vi "setSamplingMode.vi"(8 "error in (no error)":errorcluster, 10 "Fs Mode":T1, 11 "Instrument.Lockin in":refnum<class "Instrument.Lockin.lvclass">) -> (0 "error out":errorcluster, 3 "Instrument.Lockin out":refnum<class "Instrument.Lockin.lvclass">)   [LabVIEW 2019, in "Instrument.Lockin.lvclass"]
doc: "API to put lockin into IV mode.\n\nIf address=\"\", this API reads from localhost\nIf address is remote lockin, you need to add this computer to allowed whitelist on the lockin computer you are trying to access."
uses:
  Instrument.Lockin.lvclass
  Instrument.DAQ/Typedefs/DAQ.Sampling.Fs Mode--enum.ctl
  C:/Program Files (x86)/National Instruments/LabVIEW 2019/user.lib/LevyLab/Instrument Framework/SMOs/Instrument/Instrument.lvclass
  Typedefs/API/Lockin.Commands--Enum.ctl
  <userlib>/LevyLab/Instrument Framework/SMOs/Instrument/Instrument.lvclass/Instrument.ctl
  08458c74-1ef2-45d6-87a0-b6580aa97565.vi
  08458c74-1ef2-45d6-87a0-b6580aa97565.vi/21b8891c-77eb-44a0-bd46-0f361e5e9657.vi
  08458c74-1ef2-45d6-87a0-b6580aa97565.vi/21b8891c-77eb-44a0-bd46-0f361e5e9657.vi/e1bdb0cf-b8bc-43bb-a77e-4995ee286623.vi
  <userlib>/LevyLab/Instrument Framework/SMOs/Instrument/API/Send and Receive.vi
  08458c74-1ef2-45d6-87a0-b6580aa97565.vi/21b8891c-77eb-44a0-bd46-0f361e5e9657.vi/e1bdb0cf-b8bc-43bb-a77e-4995ee286623.vi/20487861-9e4a-4482-b9dd-50cdbc220220.vi
  08458c74-1ef2-45d6-87a0-b6580aa97565.vi/21b8891c-77eb-44a0-bd46-0f361e5e9657.vi/e1bdb0cf-b8bc-43bb-a77e-4995ee286623.vi/4cee38ad-58a0-4b80-9555-58bac0eb7f27.vi
  <userlib>/LevyLab/Instrument Framework/SMOs/Instrument/API/Enum to String.vi
  <userlib>/LevyLab/Instrument Framework/SMOs/RemoteControl/API/Send and Receive.vi
  <vilib>/Utility/Data Type/Get Type Information.vi
  <vilib>/JDP Science/JSONtext/JSON text to Variant.vi
  <vilib>/JDP Science/JSONtext/LVClass Serializer/JSONtext LVClass Serializer.lvclass
  Instrument.DAQ/Instrument.DAQ.lvclass
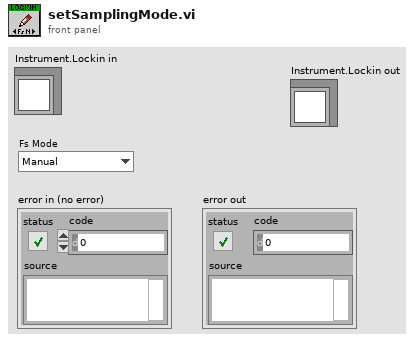
[diagram p1: front panel]
types:
  T1 = typedef "Instrument.DAQ.lvclass/DAQ.Sampling.Fs Mode--enum.ctl" = enum16{"Manual", "Auto Fs", "Max Fs"}
  T2 = typedef "Instrument.Lockin.lvclass/Lockin.Commands--Enum.ctl" = enum16{"setAI", "setAO", "setAO_Amplitude", "setAO_DC", "setAO_Frequency", "setAO_Phase", "setAO_Function", "setAO_I+", "setREF", "setREF_Frequency", "setREF_Phase", "setREF_TC", "setREF_Roll-Off", "setDAQ", "setSampling", "setOffset", "setState", "getState", "getAO", "getAI", "getResults", "getSampling", "getAOconfig", "getREFconfig", "setInputGain", "setOutputGain", "getInputGain", "getOutputGain", "setSamplingMode", "getSamplingMode", "setSweep", "getStatus", "getSweepResults", "getSweepWaveforms", "startSweep", "stopSweep", "setAUX", "getAUX"}
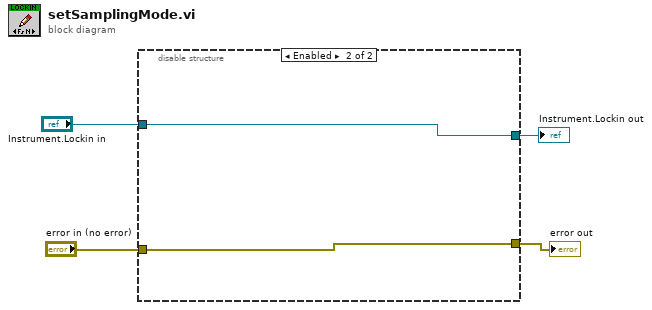
[diagram p0: block diagram]
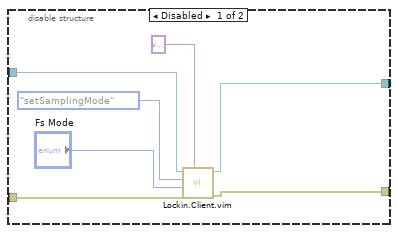
[diagram p2: hidden frame]
diagram:
  n1 = disable-structure shown="Enabled" {
    disable-tunnel: [w8 w13] -> w4
    disable-tunnel: [w7 w12] -> w3
    disable-tunnel: "Instrument.Lockin in" -> [w5 w13]
    disable-tunnel: "error in (no error)" -> [w6 w12]
    frame Disabled {
      n2 = call "Lockin.Client.vim"("Data Out type"=variant, "error in (no error)"=w6, "Data"="Fs Mode", "Command"=Lockin.Commands--Enum."setSamplingMode", "Instrument.Lockin in"=w5) -> ("error out"=w7:errorcluster, "Instrument.Lockin out"=w8:refnum<class "Instrument.Lockin.lvclass">)  [unwired: 4 in, 1 out]
    }
    frame Enabled {
    }
  }
  "Instrument.Lockin out" <- w4
  "error out" <- w3
